vi "Zero.vi"(8 "error in":errorcluster, 11 "GFG Refnum":refnum<vi>) -> (0 "error out":errorcluster, 3 "GFG Refnum Out":refnum<vi>)   [LabVIEW 2012, in "Sciscan Scope Daemon.lvlib"]
uses:
  Sciscan Scope Daemon.lvlib
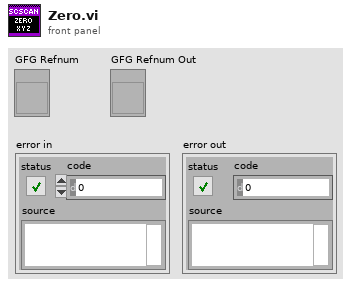
[diagram p1: front panel]
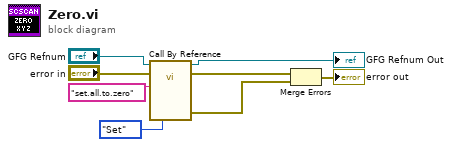
[diagram p0: block diagram]
diagram:
  n1 = call-by-ref "?"(reference="GFG Refnum", error in="error in", "Variable Name in"="set.all.to.zero", "Action"=enum16{"Init", "Set", "Get"}."Set") -> (reference out=→"GFG Refnum Out":refnum<vi>, error out=w2:errorcluster, 19:"error out"=w3:errorcluster)  [unwired: 11 in, 6 out]
  n2 = Merge Errors(w2, w3) -> (→"error out":errorcluster)
